vi "Find_Error_Bar_Data.vi"(1 "Ch Index":i32, 2 "Row Numbers":i32[](array[numeric]), 3 "Channel Values":string[][](array[string])) -> (0 "Error bar values":string[](array[string]))   [LabVIEW 2016]
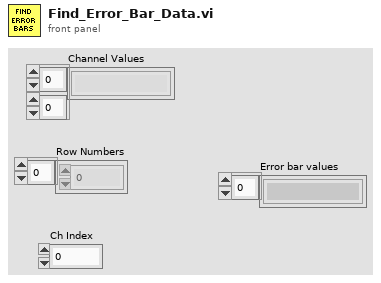
[diagram p1: front panel]
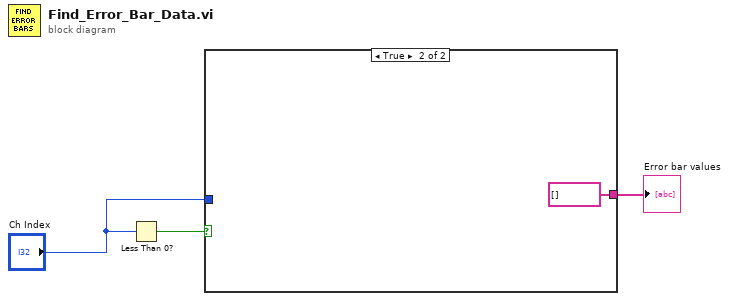
[diagram p0: block diagram]
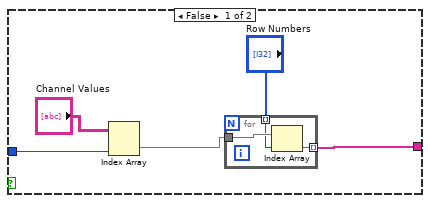
[diagram p2: hidden frame]
diagram:
  n1 = Less Than 0?(x="Ch Index") -> (x < 0?=w1:bool)
  n2 = case shown="True" w1 {
    tunnel: [w7 string[] []] -> w3
    tunnel: "Ch Index" -> [w4 _]
    frame False {
      n3 = Index Array(array="Channel Values", index (col)=w4) -> (element=w6:string[])  [unwired: 1 in]
      n4 = for {
        tunnel: w6 -> [w11]
        tunnel: "Row Numbers" -> [w10] mode=indexing
        tunnel: [w9] -> w7 mode=indexing
        n5 = Index Array(array=w11, index=w10) -> (element=w9:string)
      }
    }
    frame True {
    }
  }
  "Error bar values" <- w3
